vi "test6-ChainNodeExitSequenceCheck.vi"(8 "error in (no error)":errorcluster, 11 "TestCase in":refnum<class "testcase-CSMChainMode.lvclass">) -> (0 "error out":errorcluster, 3 "TestCase out":refnum<class "testcase-CSMChainMode.lvclass">)   [LabVIEW 2017, in "testcase-CSMChainMode.lvclass"]
uses:
  testcase-CSMChainMode.lvclass
  <vilib>/addons/_JKI Toolkits/VI Tester/TestCase.llb/TestCase.lvclass
  src/user.lib/_NEVSTOP/Communicable State Machine(CSM)/Communicable State Machine.lvlib
  CSM/CSM-Testcase.lvlib
  C:/Program Files (x86)/National Instruments/LabVIEW 2017/vi.lib/addons/_JKI Toolkits/VI Tester/TestCase.llb/TestCase.lvclass
panel:
  out "Loop Count":i32
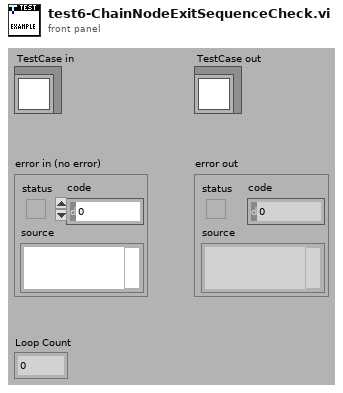
[diagram p1: front panel]
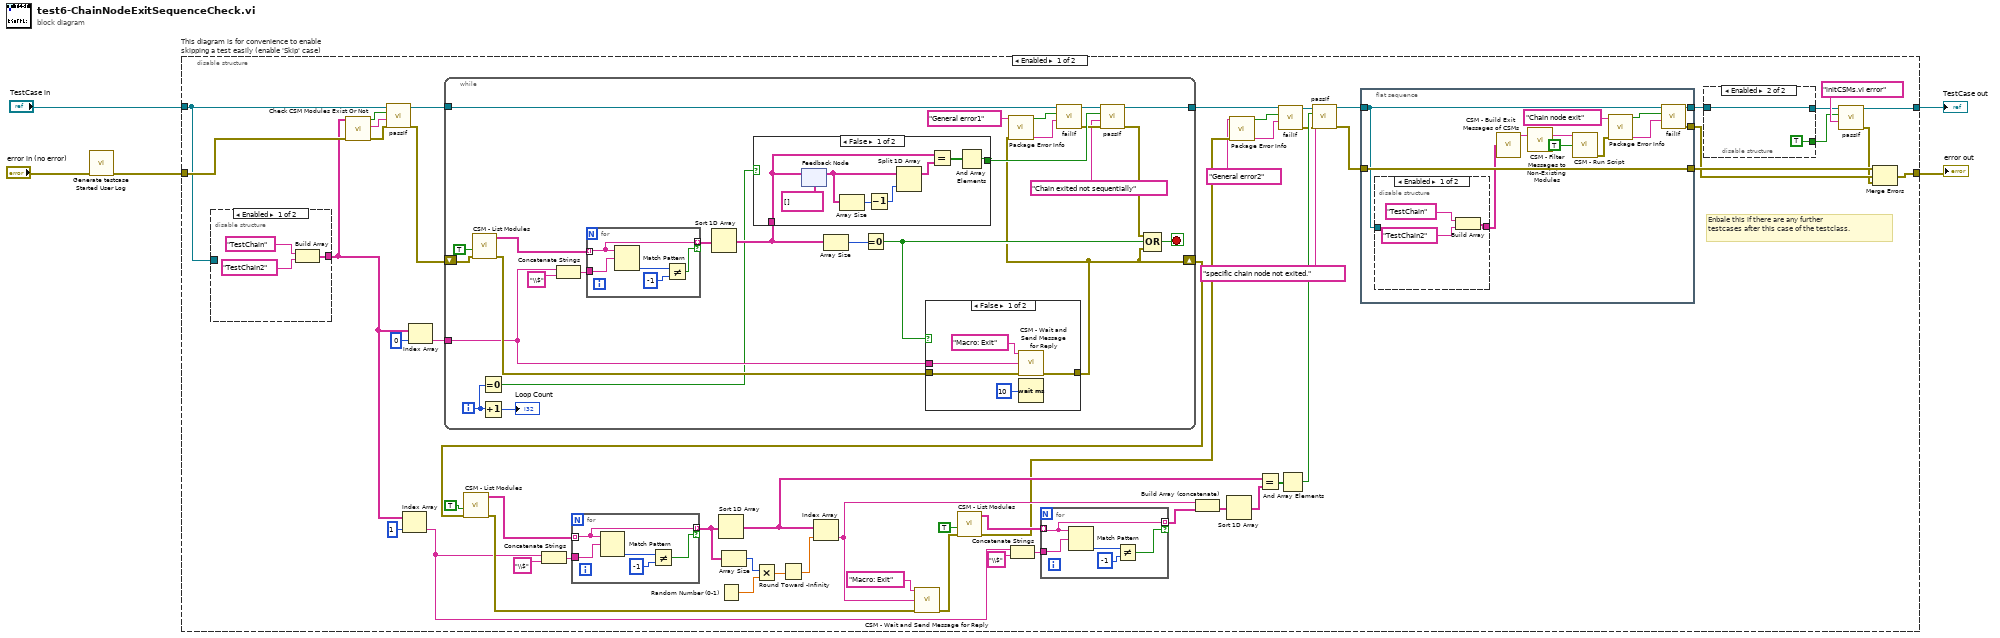
[diagram p0: block diagram]
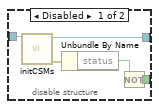
[diagram p2: hidden frame]
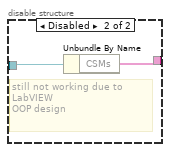
[diagram p3: hidden frame]
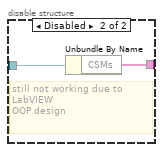
[diagram p4: hidden frame]
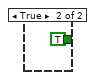
[diagram p6: hidden frame]
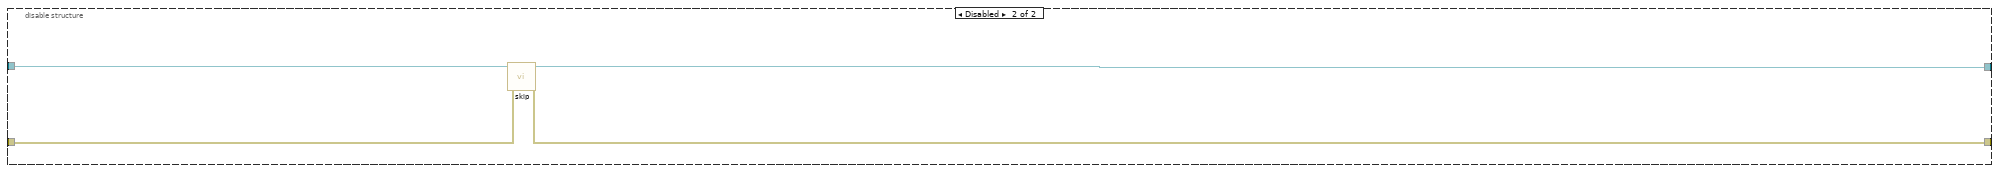
[diagram p7: hidden frame]
diagram:
  n1 = call "Generate testcase Started User Log.vi"("Error In"="error in (no error)") -> ("error out"=w1:errorcluster)  [unwired: 10 in]
  n2 = disable-structure "This diagram is for convenience to enable skipping a test easily (enable 'Skip' case)" shown="Enabled" {
    disable-tunnel: "TestCase in" -> [w6 w149]
    disable-tunnel: [w12 w147] -> w2
    disable-tunnel: [w11 w148] -> w4
    disable-tunnel: w1 -> [w26 w146]
    frame Enabled {
      # "Enbale this if there are any further\ntestcases after this case of the testclass."
      n3 = disable-structure shown="Enabled" {
        disable-tunnel: [w68 w71] -> w7
        disable-tunnel: w6 -> [_ w72]
        frame Enabled {
          n4 = Build Array("TestChain" ("CSM Name"), "TestChain2" ("CSM Name")) -> (w68:string[])
        }
        frame Disabled {
          # "still not working due to \nLabVIEW\nOOP design"
          n5 = Unbundle By Name(w72) -> ("CSMs"=w71:string[])
        }
      }
      n6 = call "Check CSM Modules Exist Or Not.vi"("error in"=w26, "CSM names in"=w7) -> ("error out"=w28:errorcluster, "Debug string"=w29:string, "All Modules Exist?"=w30:bool)  [unwired: 7 in]
      n7 = call-dynamic "passIf.vi"("error in (no error)"=w28, "message (\"\")"=w29, "pass"=w30, "TestCase in"=w6) -> ("error out"=w25:errorcluster, "TestCase out"=w27:refnum<class "testcase-CSMChainMode.lvclass">)  [unwired: 6 in]
      n8 = Index Array(array=w7, index=1) -> (element=w41:string)
      n9 = Index Array(array=w7, index=0) -> (element=w59:string)
      n10 = while {
        tunnel: w59 -> [w119]
        tunnel: w27 -> [w106]
        tunnel: [w118] -> w21
        shift-right: [w102] -> w24
        shift-left: w25 -> [w115]
        i -> [w113]
        stop <- w117 stop-if-true
        n11 = call "CSM - List Modules.vi"("Error In"=w115, "With Nodes? (F)"=TRUE) -> ("error out"=w120:errorcluster, "Module Names"=w122:string[])  [unwired: 8 in]
        n12 = Equal To 0?(x=w113) -> (x = 0?=w110:bool)
        n13 = Increment(x=w113) -> (x+1=→"Loop Count":i32)
        n14 = Concatenate Strings(w119, "\\$" ("string")) -> (w125:string)
        n15 = for {
          tunnel: w122 -> [w143] mode=indexing
          tunnel: [w143] -> w114 mode=indexing if=w142
          tunnel: w125 -> [w141]
          n16 = Match Pattern(string=w143, regular expression=w141) -> (offset past match=w145:i32)  [unwired: 1 in, 3 out]
          n17 = Not Equal?(x=w145, y=-1) -> (x != y?=w142:bool)
        }
        n18 = Sort 1D Array(array=w114) -> (sorted array=w112:string[])
        n19 = case shown="False" w110 {
          tunnel: w112 -> [w135 _]
          tunnel: [w132 TRUE] -> w111
          frame False {
            n20 = feedback #1(string[] []) -> (w138:string[])
            n21 = feedback-in #1(w135) -> ()
            n22 = Array Size(array=w138) -> (size(s)=w137:i32)
            n23 = Decrement(x=w137) -> (x-1=w136:i32)
            n24 = Split 1D Array(array=w138, index=w136) -> (first subarray=w134:string[])  [unwired: 1 out]
            n25 = Equal?(x=w135, y=w134) -> (x = y?=w133:bool[])
            n26 = And Array Elements(Boolean array=w133) -> (logical AND=w132:bool)
          }
          frame True {
          }
        }
        n27 = Array Size(array=w112) -> (size(s)=w121:i32)
        n28 = Equal To 0?(x=w121) -> (x = 0?=w109:bool)
        n29 = case shown="False" w109 {
          tunnel: w120 -> [w130 w131]
          tunnel: w119 -> [w129 _]
          tunnel: [w127 w131] -> w102
          frame False {
            n30 = call "CSM - Wait and Send Message for Reply.vi"("State"="Macro: Exit", "Target Module"=w129, "Error In (No Error)"=w130) -> ("error out"=w127:errorcluster)  [unwired: 9 in, 3 out]
            n31 = Wait (ms)(milliseconds to wait=u32 10) -> ()  [unwired: 1 out]
          }
          frame True {
          }
        }
        n32 = call "Package Error Info.vi"("error in"=w102, "String in"="General error1") -> ("packed error info out"=w107:string, "error status"=w108:bool)  [unwired: 8 in]
        n33 = call-dynamic "failIf.vi"("message (\"\")"=w107, "fail"=w108, "TestCase in"=w106) -> ("error out"=w104:errorcluster, "TestCase out"=w105:refnum<class "testcase-CSMChainMode.lvclass">)  [unwired: 7 in]
        n34 = call-dynamic "passIf.vi"("error in (no error)"=w104, "message (\"\")"="Chain exited not sequentially" ("message (\"\")"), "pass"=w111, "TestCase in"=w105) -> ("error out"=w103:errorcluster, "TestCase out"=w118:refnum<class "testcase-CSMChainMode.lvclass">)  [unwired: 6 in]
        n35 = Compound Arithmetic op=OR(w103, w109, w102) -> (w117:bool)
      }
      n36 = call "CSM - List Modules.vi"("Error In"=w24, "With Nodes? (F)"=TRUE) -> ("error out"=w47:errorcluster, "Module Names"=w57:string[])  [unwired: 8 in]
      n37 = Concatenate Strings(w41, "\\$" ("string")) -> (w54:string)
      n38 = for {
        tunnel: w57 -> [w97] mode=indexing
        tunnel: [w97] -> w53 mode=indexing if=w96
        tunnel: w54 -> [w95]
        n39 = Match Pattern(string=w97, regular expression=w95) -> (offset past match=w99:i32)  [unwired: 1 in, 3 out]
        n40 = Not Equal?(x=w99, y=-1) -> (x != y?=w96:bool)
      }
      n41 = Sort 1D Array(array=w53) -> (sorted array=w36:string[])
      n42 = Random Number (0-1)() -> (number: 0 to 1=w51:dbl)
      n43 = Array Size(array=w53) -> (size(s)=w52:i32)
      n44 = Multiply(x=w52, y=w51) -> (x*y=w50:dbl)
      n45 = Round Toward -Infinity(1:w50) -> (0:w49:dbl)
      n46 = Index Array(array=w36, index=w49) -> (element=w39:string)
      n47 = call "CSM - Wait and Send Message for Reply.vi"("State"="Macro: Exit", "Target Module"=w39, "Error In (No Error)"=w47) -> ("error out"=w43:errorcluster)  [unwired: 9 in, 3 out]
      n48 = call "CSM - List Modules.vi"("Error In"=w43, "With Nodes? (F)"=TRUE) -> ("error out"=w18:errorcluster, "Module Names"=w42:string[])  [unwired: 8 in]
      n49 = Concatenate Strings(w41, "\\$" ("string")) -> (w46:string)
      n50 = for {
        tunnel: [w90] -> w40 mode=indexing if=w92
        tunnel: w46 -> [w91]
        tunnel: w42 -> [w90] mode=indexing
        n51 = Match Pattern(string=w90, regular expression=w91) -> (offset past match=w94:i32)  [unwired: 1 in, 3 out]
        n52 = Not Equal?(x=w94, y=-1) -> (x != y?=w92:bool)
      }
      n53 = Build Array (concatenate)(w39, w40) -> (w38:string[])
      n54 = Sort 1D Array(array=w38) -> (sorted array=w37:string[])
      n55 = call "Package Error Info.vi"("error in"=w18, "String in"="General error2") -> ("packed error info out"=w23:string, "error status"=w22:bool)  [unwired: 8 in]
      n56 = Equal?(x=w36, y=w37) -> (x = y?=w35:bool[])
      n57 = call-dynamic "failIf.vi"("message (\"\")"=w23, "fail"=w22, "TestCase in"=w21) -> ("error out"=w19:errorcluster, "TestCase out"=w20:refnum<class "testcase-CSMChainMode.lvclass">)  [unwired: 7 in]
      n58 = And Array Elements(Boolean array=w35) -> (logical AND=w34:bool)
      n59 = call-dynamic "passIf.vi"("error in (no error)"=w19, "message (\"\")"="specific chain node not exited.", "pass"=w34, "TestCase in"=w20) -> ("error out"=w31:errorcluster, "TestCase out"=w33:refnum<class "testcase-CSMChainMode.lvclass">)  [unwired: 6 in]
      n60 = flat-sequence {
        tunnel: w33 -> [w73]
        tunnel: [w78] -> w32
        tunnel: w31 -> [w81]
        tunnel: [w81] -> w10
        tunnel: [w75] -> w9
        frame #0 {
          n61 = disable-structure shown="Enabled" {
            disable-tunnel: [w85 w88] -> w74
            disable-tunnel: w73 -> [_ w89]
            frame Enabled {
              n62 = Build Array("TestChain" ("CSM Name"), "TestChain2" ("CSM Name")) -> (w85:string[])
            }
            frame Disabled {
              # "still not working due to \nLabVIEW\nOOP design"
              n63 = Unbundle By Name(w89) -> ("CSMs"=w88:string[])
            }
          }
          n64 = call "CSM - Build Exit Messages of CSMs.vi"("CSMs"=w74) -> ("States"=w83:string)  [unwired: 14 in]
          n65 = call "CSM - Filter Messages to Non-Existing Modules.vi"("States In"=w83) -> ("States Out"=w84:string)  [unwired: 14 in]
          n66 = call "CSM - Run Script.vi"("CSM Scripts"=w84, "Continue If Error? (F)"=TRUE) -> ("error out"=w77:errorcluster)  [unwired: 11 in, 2 out]
          n67 = call "Package Error Info.vi"("error in"=w77, "String in"="Chain node exit") -> ("packed error info out"=w80:string, "error status"=w79:bool)  [unwired: 8 in]
          n68 = call-dynamic "failIf.vi"("message (\"\")"=w80, "fail"=w79, "TestCase in"=w73) -> ("error out"=w75:errorcluster, "TestCase out"=w78:refnum<class "testcase-CSMChainMode.lvclass">)  [unwired: 7 in]
        }
      }
      n69 = disable-structure shown="Enabled" {
        disable-tunnel: w32 -> [w65 w67]
        disable-tunnel: [w64 TRUE ("pass")] -> w14
        disable-tunnel: [w63 w67] -> w13
        frame Disabled {
          n70 = call "initCSMs.vi"("TestCase in"=w65) -> ("error out"=w62:errorcluster, "TestCase out"=w63:refnum<class "testcase-CSMChainMode.lvclass">)  [unwired: 9 in]
          n71 = Unbundle By Name(w62) -> ("status"=w61:bool)
          n72 = Not(x=w61) -> (.not. x?=w64:bool)
        }
        frame Enabled {
        }
      }
      n73 = call-dynamic "passIf.vi"("message (\"\")"="initCSMs.vi error" ("message (\"\")"), "pass"=w14, "TestCase in"=w13) -> ("error out"=w8:errorcluster, "TestCase out"=w12:refnum<class "testcase-CSMChainMode.lvclass">)  [unwired: 7 in]
      n74 = Merge Errors(w10, w9, w8) -> (w11:errorcluster)
    }
    frame Disabled {
      # "skip test result while test is under development"
      n75 = call <vilib>:"skip.vi"("error in (no error)"=w146, "TestCase in"=w149) -> ("error out"=w148:errorcluster, "TestCase out"=w147:refnum<class "testcase-CSMChainMode.lvclass">)  [unwired: 8 in]
    }
  }
  "error out" <- w4
  "TestCase out" <- w2
